vi "RuO2 10k.vi"(1 "temperature \n(OR resistance)":dbl) -> (0 "resistance \n(OR temperature)":dbl)   [LabVIEW 2013]
panel:
  # "This tool convert data for a 10K thermometer (RuO2). Edit \nconstants in the block diagram to modify calibration."
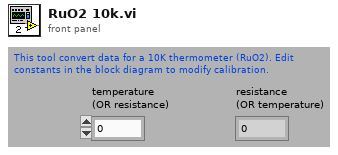
[diagram p1: front panel]
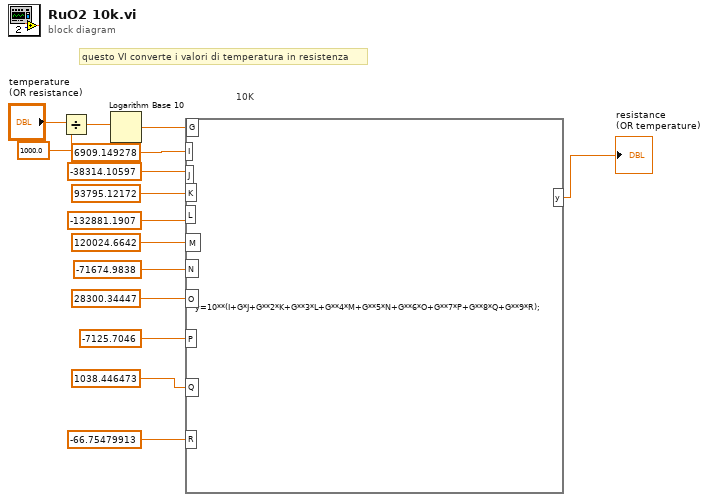
[diagram p0: block diagram]
diagram:
  # "10K"
  # "questo VI converte i valori di temperatura in resistenza"
  n1 = Divide(x="temperature \n(OR resistance)", y=1000.0) -> (x/y=w2:dbl)
  n2 = Logarithm Base 10(1:w2) -> (0:w15:dbl)
  n3 = formula code="y=10**(I+G*J+G**2*K+G**3*L+G**4*M+G**5*N+G**6*O+G**7*P+G**8*Q+G**9*R);"("G"=w15, "I"=6909.149278 ("input variable"), "L"=-132881.1907 ("input variable"), "M"=120024.6642 ("input variable"), "O"=28300.34447 ("input variable"), "Q"=1038.446473 ("input variable"), "R"=-66.75479913 ("input variable"), "P"=-7125.7046 ("input variable"), "N"=-71674.9838 ("input variable"), "J"=-38314.10597 ("input variable"), "K"=93795.12172 ("input variable")) -> ("y"=→"resistance \n(OR temperature)":dbl)
